vi "Interpolate 2D (2d X,Y).vi"(4 "ntimes":i32=1, 6 "yi":dbl[][](array[numeric]), 7 "method":i32(ring)=1 items=["nearest", "bilinear", "bicubic", "bicubic spline"], 8 "xi":dbl[][](array[numeric]), 9 "Y":dbl[][](array[numeric]), 10 "X":dbl[][](array[numeric]), 11 "Z":dbl[][](array[numeric])) -> (0 "error":i32, 1 "yi used":dbl[][](array[numeric]), 2 "xi used":dbl[][](array[numeric]), 3 "zi":dbl[][](array[numeric]))   [LabVIEW 2014, in "NI_Gmath.lvlib"]
doc: "Performs two-dimensional interpolation using a selected interpolation method based on the lookup table defined by <B>X</B>, <B>Y</B>, and <B>Z</B>, where <B>Z</B> is a 2D array. You must manually select the polymorphic instance to use."
uses:
  NI_Gmath.lvlib
panel:
  # "Interpolate 2D (2d X,Y)"
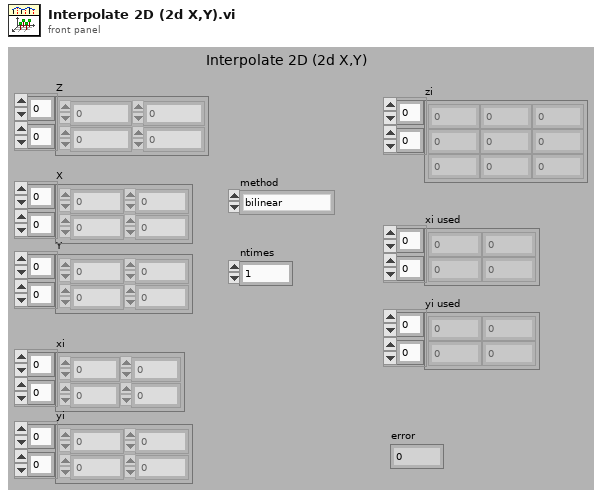
[diagram p1: front panel]
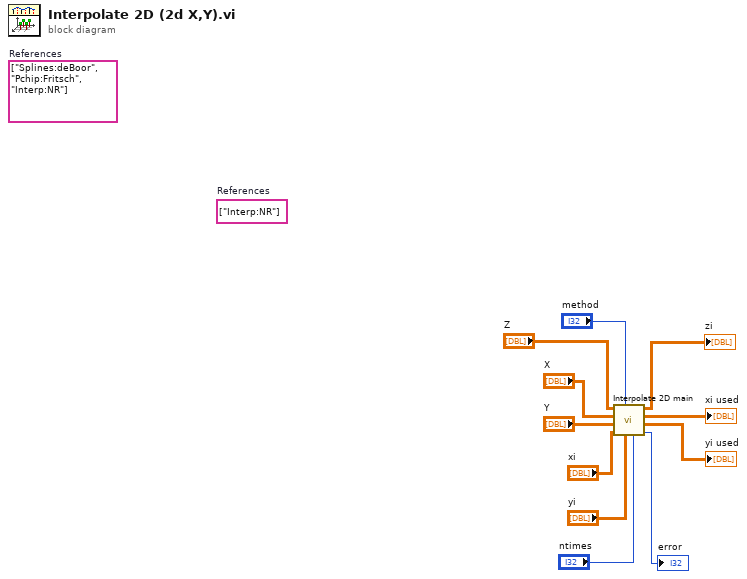
[diagram p0: block diagram]
diagram:
  (unwired) string[] ["Interp:NR"]  # References
  (unwired) string[] ["Splines:deBoor", "Pchip:Fritsch", "Interp:NR"]  # References
  n1 = call "Interpolate 2D main.vi"("ntimes"="ntimes", "yi"="yi", "method"="method", "xi"="xi", "Y"="Y", "X"="X", "Z"="Z") -> ("error"=→"error":i32, "yi used"=→"yi used":dbl[][], "xi used"=→"xi used":dbl[][], "zi"=→"zi":dbl[][])  [unwired: 1 in]
